vi "niRFUtil CONV Number to 2n.vi"(3 "Number":dbl format="%.2f") -> (0 "2^n Lower Value":i32, 1 "2^n Upper Value":i32)   [LabVIEW 2015, in "niRFUtil.lvlib"]
doc: "(c) Copyright 2006, National Instruments, Inc. This VI may not be duplicated, sold, or distributed without written consent from National Instruments."
uses:
  niRFUtil.lvlib
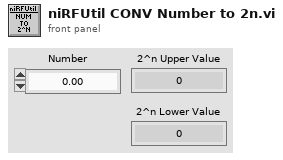
[diagram p1: front panel]
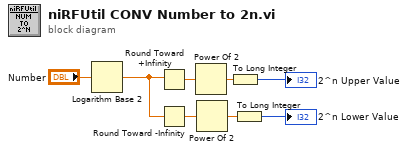
[diagram p0: block diagram]
diagram:
  n1 = Logarithm Base 2(1:"Number") -> (0:w7:dbl)
  n2 = Round Toward +Infinity(x=w7) -> (ceil(x): smallest int >= x=w6:dbl)
  n3 = Round Toward -Infinity(1:w7) -> (0:w5:dbl)
  n4 = Power Of 2(x=w6) -> (2^x=w4:dbl)
  n5 = Power Of 2(x=w5) -> (2^x=w3:dbl)
  n6 = To Long Integer(number=w4) -> (32bit integer=→"2^n Upper Value":i32)
  n7 = To Long Integer(number=w3) -> (32bit integer=→"2^n Lower Value":i32)
